vi "Set Language.vi"(8 "error in (no error)":errorcluster, 10 "Chinese?":bool, 11 "Handle in":i32) -> (0 "error out":errorcluster, 3 "Handle out":i32)   [LabVIEW 2013, in "Thorlabs_MC2000B.lvlib"]
doc: "Set display language (F: English, T: Chinese)."
uses:
  <instrlib>/Thorlabs_MC2000B/Thorlabs_MC2000B.lvlib
  Program Files/National Instruments/LabVIEW 2011/instr.lib/Thorlabs_MC2000B/Library/MC2000CommandLibWin64.dll
  <instrlib>/Thorlabs_MC2000B/Library/MC2000CommandLibWin32.dll
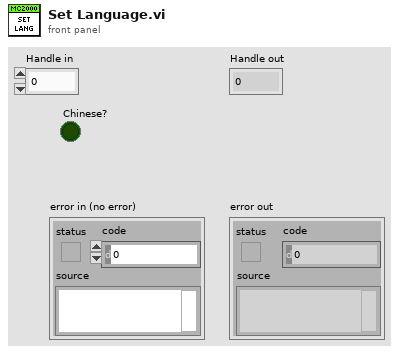
[diagram p1: front panel]
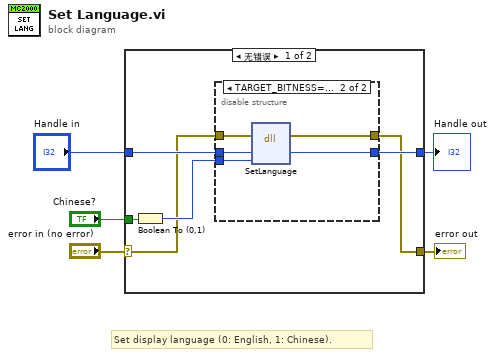
[diagram p0: block diagram]
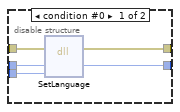
[diagram p2: hidden frame]
diagram:
  # "Set display language (0: English, 1: Chinese)."
  n1 = case shown="无错误" "error in (no error)" {
    selector: "error in (no error)" -> [w7 w23]
    tunnel: [w6 w23] -> w5
    tunnel: "Chinese?" -> [w9 _]
    tunnel: "Handle in" -> [w11 w22]
    tunnel: [w10 w22] -> w1
    frame No Error {
      n2 = Boolean To (0,1)(Boolean=w9) -> (0, 1=w8:i16)
      n3 = disable-structure shown="TARGET_BITNESS==32" {
        disable-tunnel: w11 -> [w16 w21]
        disable-tunnel: [w15 w20] -> w10
        disable-tunnel: w8 -> [w14 w19]
        disable-tunnel: w7 -> [w13 w18]
        disable-tunnel: [w12 w17] -> w6
        frame condition #0 {
          n4 = dll-call lib="D:/Program Files/National Instruments/LabVIEW 2011/instr.lib/Thorlabs_MC2000B/Library/MC2000CommandLibWin64.dll" fn="SetLanguage"(error in=w13, "hdl"=w16, "language"=w14) -> (error out=w12:errorcluster, "hdl"=w15:i32)  [unwired: 4 in, 1 out]
        }
        frame condition #1 (active) {
          n5 = dll-call lib="C:/Program Files (x86)/National Instruments/LabVIEW 2013/instr.lib/Thorlabs_MC2000B/Library/MC2000CommandLibWin32.dll" fn="SetLanguage"(error in=w18, "hdl"=w21, "language"=w19) -> (error out=w17:errorcluster, "hdl"=w20:i32)  [unwired: 4 in, 1 out]
        }
      }
    }
    frame Error {
    }
  }
  "error out" <- w5
  "Handle out" <- w1
